vi "XIPIN_Viterbi_Decoder_7_0.vi"   [LabVIEW 2017]
doc: "The Xilinx Viterbi Decoder LogiCORE is fully synchronous, using a single clock. Options include parameterizable constraint length, convolutional codes and traceback length. Various architectures are available including parallel, serial, multi-channel and dual decoding. The core is delivered through the Xilinx CORE Generator System and integrates seamlessly with the Xilinx design flow.\n------------------------------------\n<b>Need License</b> : Yes"
uses:
  <vilib>/rvi/XilinxIP/XIPIN_XNode/niFpgaXIPIN.xnode
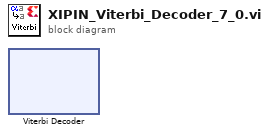
[diagram p0: block diagram]
diagram:
  n1 = xnode ("Viterbi Decoder")() -> ()
